vi "Variants equal.vi"(1 "Variant 2":variant, 2 "Variant 1":variant) -> (0 "Same?":bool)   [LabVIEW 2011]
doc: "Returns true if inputs are equal.\n\n\nVersion 1.0 - 02/27/2013\n\nPhaeron, Inc.\nwww.phaeron.com\ninfo@phaeron.com"
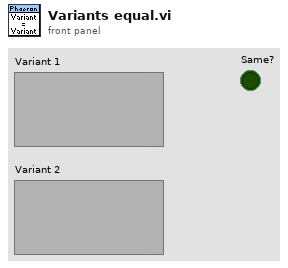
[diagram p1: front panel]
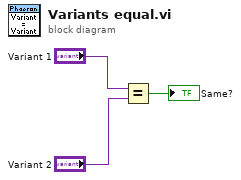
[diagram p0: block diagram]
diagram:
  n1 = Equal?(x="Variant 1", y="Variant 2") -> (x = y?=→"Same?":bool)
